vi "ArgType_to_String.vi"(4 "arg type":T1) -> (1 "arg type string":string)   [LabVIEW 2016, in "PyLVi.lvlib" / "PyLVi.lvclass"]
uses:
  PyLVi.lvclass
  Controls/ArgumentType.ctl
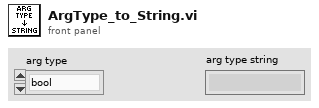
[diagram p1: front panel]
types:
  T1 = typedef "PyLVi.lvlib/PyLVi.lvclass/ArgumentType.ctl" = enum8{"bool", "numeric", "string", "dict", "ndarray", "ndarray2d"}
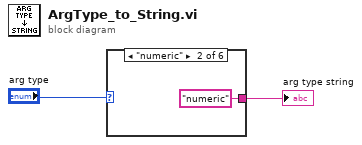
[diagram p0: block diagram]
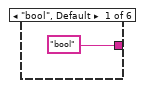
[diagram p2: hidden frame]
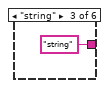
[diagram p3: hidden frame]
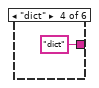
[diagram p4: hidden frame]
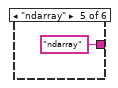
[diagram p5: hidden frame]
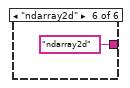
[diagram p6: hidden frame]
diagram:
  n1 = case shown="\"numeric\"" "arg type" {
    tunnel: ["bool" ("data type string") "numeric" ("data type string") "string" ("data type string") "dict" ("data type string") "ndarray" ("data type string") "ndarray2d" ("data type string")] -> w1
    frame "bool", Default {
    }
    frame "numeric" {
    }
    frame "string" {
    }
    frame "dict" {
    }
    frame "ndarray" {
    }
    frame "ndarray2d" {
    }
  }
  "arg type string" <- w1
